vi "Goodbye (async).vi"(9 "Goodbye Request":T1={"Error URI"="wamp.close.shut_down", "Message"="client disconnect"}, 10 "error in (no error)":errorcluster, 11 "WAMP Client in":refnum<class "WAMP Client.lvclass">) -> (2 "error out":errorcluster, 3 "WAMP Client out":refnum<class "WAMP Client.lvclass">)   [LabVIEW 2020, in "WAMP Client.lvclass"]
uses:
  <userlib>/lvwamp/WAMP Client/WAMP Client.lvclass
  <userlib>/lvwamp/WAMP Client/TypeDef/GOODBYE Request Data.ctl
  <userlib>/lvwamp/WAMP Client/TypeDef/Internal Message Type.ctl
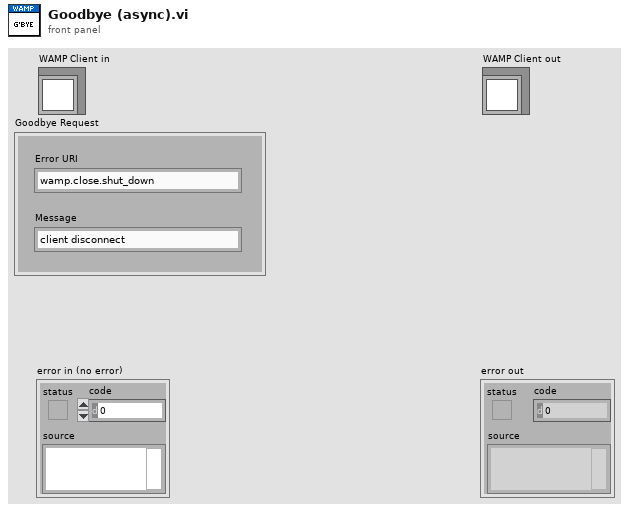
[diagram p1: front panel]
types:
  T1 = typedef "WAMP Client.lvclass/GOODBYE Request Data.ctl" = cluster{"Error URI":string, "Message":string}
  T2 = typedef "WAMP Client.lvclass/Internal Message Type.ctl" = enum16{"Subscribe", "Handle Subscribed", "Handle Event", "Unsubscribe", "Handle Unsubscribed", "Publish", "Handled Published", "Goodbye", "Handle Goodbye", "Call", "Handle Result"}
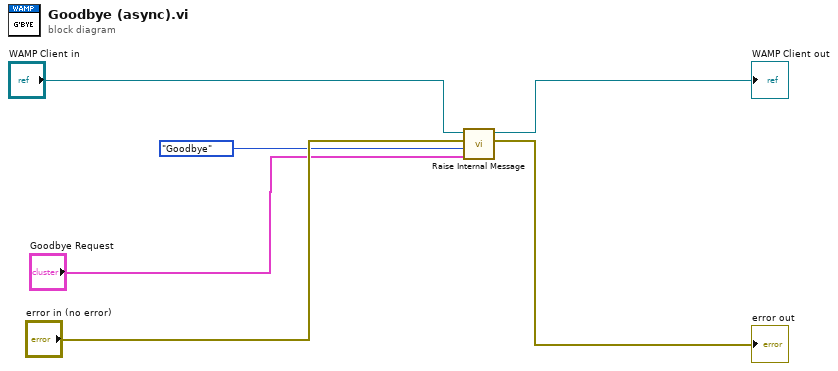
[diagram p0: block diagram]
diagram:
  n1 = call-dynamic "Raise Internal Message.vi"("Variant"="Goodbye Request", "Internal Message Type"=Internal_Message_Type."Goodbye", "error in (no error)"="error in (no error)", "WAMP Client in"="WAMP Client in") -> ("error out"=→"error out":errorcluster, "WAMP Client out"=→"WAMP Client out":refnum<class "WAMP Client.lvclass">)  [unwired: 6 in]
